vi "Array with For Loop.vi"() -> ()   [LabVIEW 2023]
panel:
  out "number: 0 to 1":dbl
  out "Array":dbl[](array[numeric])
  in  "Numeric 2":i32
  out "Numeric":i32
  out "number (0 to 1)":dbl
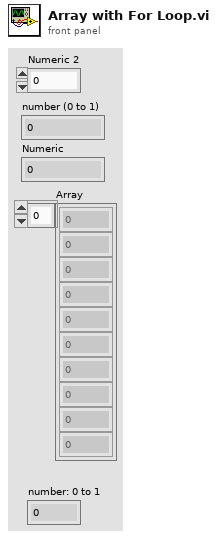
[diagram p1: front panel]
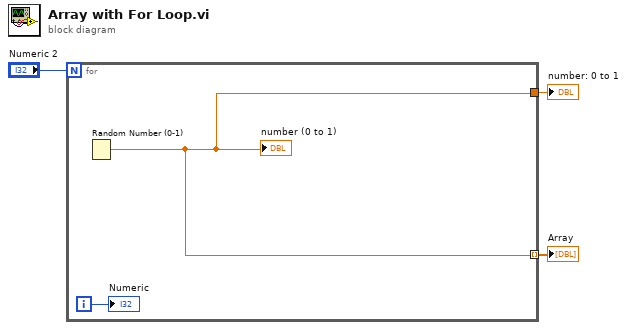
[diagram p0: block diagram]
diagram:
  n1 = for {
    N: "Numeric 2" -> [_]
    tunnel: [w4] -> w2 mode=indexing
    tunnel: [w4] -> w1
    i -> [w5]
    n2 = Random Number (0-1)() -> (number: 0 to 1=w4:dbl)
    "number (0 to 1)" <- w4
    "Numeric" <- w5
  }
  "Array" <- w2
  "number: 0 to 1" <- w1
